vi "Create Public User Events.vi"(8 "error in (no error)":errorcluster, 11 "TwinCAT ADS in":refnum<class "TwinCAT ADS.lvclass">) -> (0 "error out":errorcluster, 3 "TwinCAT ADS out":refnum<class "TwinCAT ADS.lvclass">)   [LabVIEW 2018, in "TwinCAT ADS.lvclass"]
uses:
  TwinCAT ADS.lvclass
  Controls/Connection State Change Event Data.ctl
  Controls/ADS Notification Event Data.ctl
  Controls/Symbol Information.ctl
  Controls/AMS Router Notification Event Data.ctl
  Controls/AMS Router State.ctl
  Controls/State Information.ctl
  TwinCAT ADS.lvclass/TwinCAT ADS.ctl
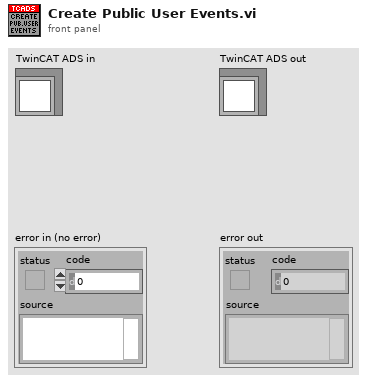
[diagram p1: front panel]
types:
  T1 = typedef "TwinCAT ADS.lvclass/Connection State Change Event Data.ctl" = cluster{"Old State":enum16{"None, Unknown", "Disconnected", "Connected", "Lost"}, "New State":enum16{"None, Unknown", "Disconnected", "Connected", "Lost"}, "Reason":enum16{"None", "Established", "Closed", "Lost", "Error", "Resurrected"}}
  T2 = typedef "TwinCAT ADS.lvclass/ADS Notification Event Data.ctl" = cluster{"Alias":string, "Symbol Info":T3, "Value":variant}
  T3 = typedef "TwinCAT ADS.lvclass/Symbol Information.ctl" = cluster{"Name":string, "Short Name":string, "Size":i32, "Type Category":i32, "Type Name":string, "Type ID":i32, "Index Group":i64, "Index Offset":i64, "Child Count":i32, "Has Rpc Methods?":bool, "Comment":string}
  T4 = typedef "TwinCAT ADS.lvclass/AMS Router Notification Event Data.ctl" = cluster{"State":T5}
  T5 = typedef "TwinCAT ADS.lvclass/AMS Router State.ctl" = enum32{"Stop", "Start", "Removed", "Unknown"}
  T6 = typedef "TwinCAT ADS.lvclass/State Information.ctl" = cluster{"ADS State":enum16{"Invalid", "Idle", "Reset", "Init", "Start", "Run", "Stop", "SaveConfig", "LoadConfig", "PowerFailure", "PowerGood", "Error", "Shutdown", "Suspend", "Resume", "Config", "Reconfig", "Stopping, Maxstates", "Incompatible", "Exception"}, "Device State":i16}
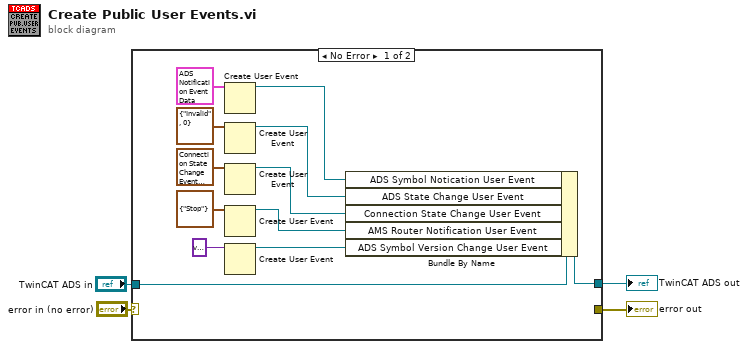
[diagram p0: block diagram]
diagram:
  n1 = case shown="No Error" "error in (no error)" {
    selector: "error in (no error)" -> [_ w17]
    tunnel: "TwinCAT ADS in" -> [w11 w18]
    tunnel: [w6 w18] -> w3
    tunnel: [_ w17] -> w1
    frame No Error {
      n2 = Create User Event(user event datatype=T2 {"Alias"="", "Symbol Info"={"Name"="", "Short Name"="", "Size"=0, "Type Category"=0, "Type Name"="", "Type ID"=0, "Index Group"=0, "Index Offset"=0, "Child Count"=0, "Has Rpc Methods?"=FALSE, "Comment"=""}, "Value"=variant} ("TwinCAT ADS.Symbol Notification")) -> (user event=w10:refnum<user-event>)  [unwired: 1 in, 1 out]
      n3 = Create User Event(user event datatype=T6 {"ADS State"=enum."Invalid", "Device State"=0} ("TwinCAT ADS.State Change")) -> (user event=w9:refnum<user-event>)  [unwired: 1 in, 1 out]
      n4 = Create User Event(user event datatype=T1 {"Old State"=enum."None, Unknown", "New State"=enum."None, Unknown", "Reason"=enum."None"} ("TwinCAT ADS.Connection State Change")) -> (user event=w8:refnum<user-event>)  [unwired: 1 in, 1 out]
      n5 = Create User Event(user event datatype=T4 {"State"=enum."Stop"} ("TwinCAT ADS.AMS Router Notification")) -> (user event=w7:refnum<user-event>)  [unwired: 1 in, 1 out]
      n6 = Create User Event(user event datatype=variant ("Void")) -> (user event=w5:refnum<user-event>)  [unwired: 1 in, 1 out]
      n7 = Bundle By Name(cluster=w11, "ADS Symbol Notication User Event"=w10, "ADS State Change User Event"=w9, "Connection State Change User Event"=w8, "AMS Router Notification User Event"=w7, "ADS Symbol Version Change User Event"=w5) -> (w6:refnum<class "TwinCAT ADS.lvclass">)
    }
    frame Error {
    }
  }
  "error out" <- w1
  "TwinCAT ADS out" <- w3
